vi "Write String to Log File.vi"(9 "operation (Open or Create)":T1(ring)=enum."open or create", 10 "string to log":string, 11 "log file":path=path "c:/ni-rt/VeriStand/Custom Devices/CD debug log.txt") -> (0 "error out":errorcluster)   [LabVIEW 2020]
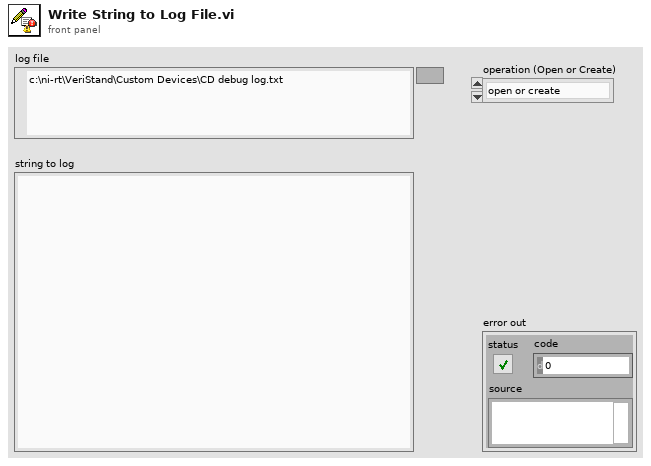
[diagram p1: front panel]
types:
  T1 = enum16{"open", "replace", "create", "open or create", "replace or create", "replace or create with confirmation"}
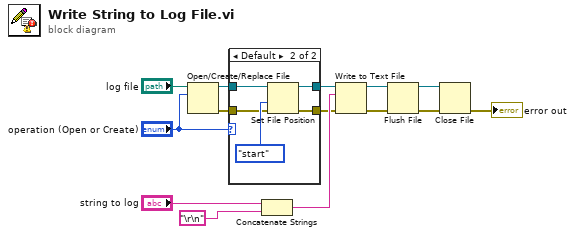
[diagram p0: block diagram]
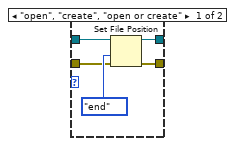
[diagram p2: hidden frame]
diagram:
  n1 = Open/Create/Replace File(file path (use dialog)="log file", operation (0:open)="operation (Open or Create)") -> (refnum out=w6:refnum<file>, error out=w5:errorcluster)  [unwired: 4 in, 1 out]
  n2 = case shown="Default" "operation (Open or Create)" {
    tunnel: w6 -> [w18 w23]
    tunnel: w5 -> [w17 w22]
    tunnel: [w16 w21] -> w4
    tunnel: [w15 w20] -> w3
    frame "open", "create", "open or create" {
      n3 = Set File Position(refnum=w18, from (0:start)=enum16{"start", "end", "current"}."end", error in=w17) -> (refnum out=w15:refnum<file>, error out=w16:errorcluster)  [unwired: 1 in]
    }
    frame Default {
      n4 = Set File Position(refnum=w23, from (0:start)=enum16{"start", "end", "current"}."start", error in=w22) -> (refnum out=w20:refnum<file>, error out=w21:errorcluster)  [unwired: 1 in]
    }
  }
  n5 = Concatenate Strings("string to log", "\r\n" ("string")) -> (w11:string)
  n6 = Write to Text File(file (use dialog)=w3, text=w11, error in=w4) -> (refnum out=w9:refnum<file>, error out=w10:errorcluster)  [unwired: 1 in, 1 out]
  n7 = Flush File(refnum=w9, error in=w10) -> (refnum out=w8:refnum<file>, error out=w7:errorcluster)
  n8 = Close File(refnum=w8, error in=w7) -> (error out=→"error out":errorcluster)  [unwired: 1 out]
